vi "Test Set Class.vi"(8 "error in (no error)":errorcluster, 11 "TestCase in":refnum<class "Test FP.lvclass">) -> (0 "error out":errorcluster, 3 "TestCase out":refnum<class "Test FP.lvclass">)   [LabVIEW 2020, in "Test FP.lvclass"]
uses:
  Test FP.lvclass
  Classes/Implementations/Osciloscope/Osciloscope.lvclass
  <vilib>/addons/_JKI Toolkits/VI Tester/TestCase.llb/TestCase.lvclass
  C:/Program Files (x86)/National Instruments/LabVIEW 2020/vi.lib/addons/_JKI Toolkits/VI Tester/TestCase.llb/TestCase.lvclass
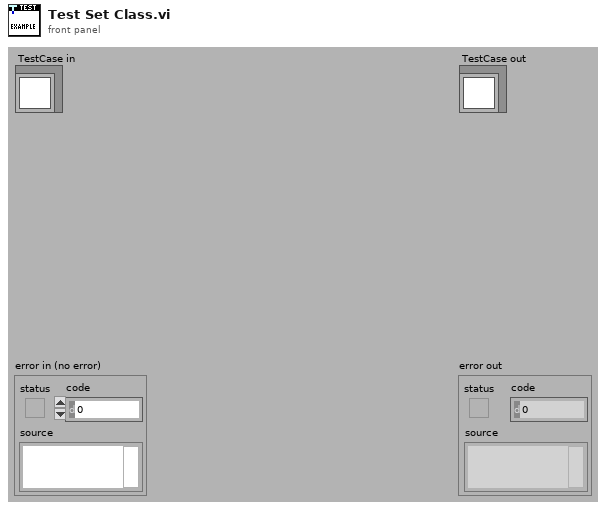
[diagram p1: front panel]
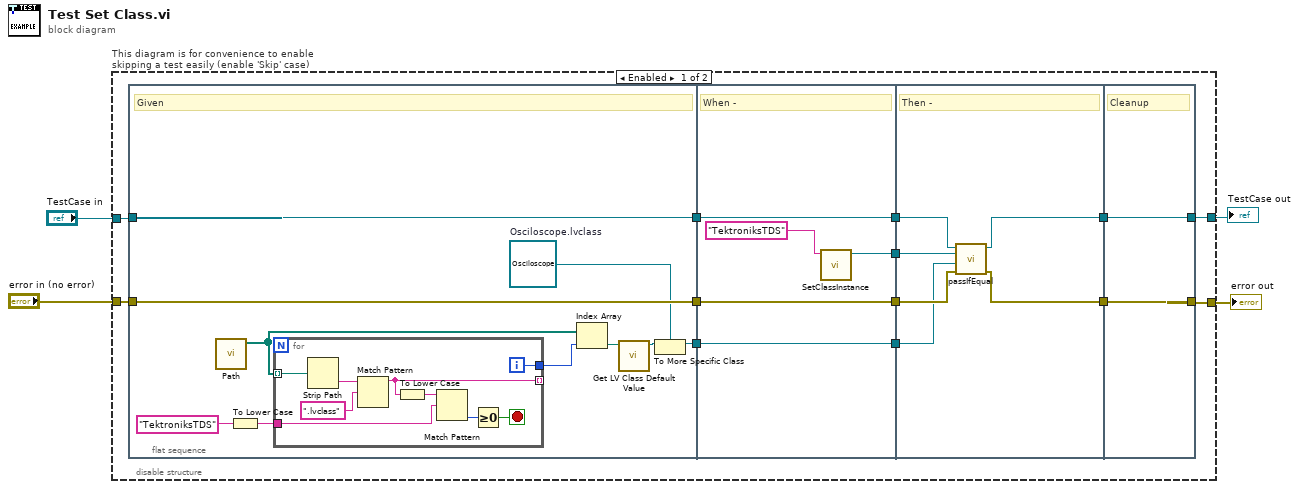
[diagram p0: block diagram]
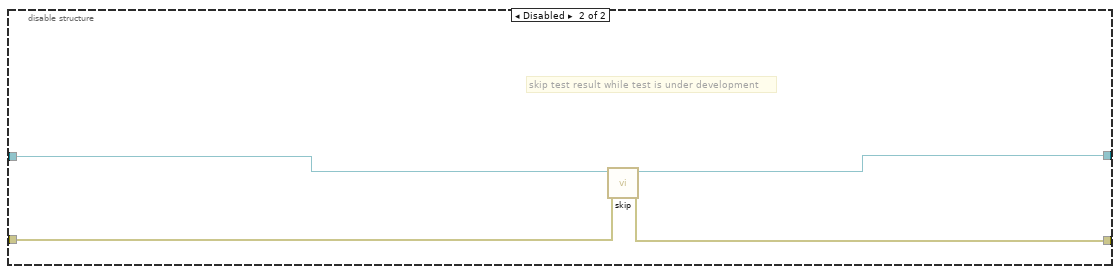
[diagram p2: hidden frame]
diagram:
  n1 = disable-structure "This diagram is for convenience to enable skipping a test easily (enable 'Skip' case)" shown="Enabled" {
    disable-tunnel: "TestCase in" -> [w11 w53]
    disable-tunnel: [w9 w51] -> w1
    disable-tunnel: [w8 w52] -> w3
    disable-tunnel: "error in (no error)" -> [w10 w50]
    frame Enabled {
      n2 = flat-sequence {
        tunnel: w10 -> [w26]
        tunnel: w11 -> [w27]
        tunnel: [w27] -> w17
        tunnel: [w26] -> w16
        tunnel: [w18] -> w5
        tunnel: [w41] -> w15
        tunnel: [w40] -> w14
        tunnel: w17 -> [w41]
        tunnel: w16 -> [w40]
        tunnel: [w39] -> w7
        tunnel: [w38] -> w6
        tunnel: w5 -> [w38]
        tunnel: [w46] -> w13
        tunnel: [w44] -> w12
        tunnel: w15 -> [w47]
        tunnel: w14 -> [w45]
        tunnel: w7 -> [w43]
        tunnel: w6 -> [w42]
        tunnel: [w48] -> w8
        tunnel: [w49] -> w9
        tunnel: w13 -> [w49]
        tunnel: w12 -> [w48]
        frame #0 {
          w21 = refnum<class "Osciloscope.lvclass"> refnum  # Osciloscope.lvclass
          # "Given"
          n3 = call "Path.vi"() -> ("All Files in Dir"=w19:path[])  [unwired: 11 in]
          n4 = To Lower Case(string="TektroniksTDS") -> (all lower case string=w25:string)
          n5 = for {
            tunnel: w19 -> [w35] mode=indexing
            tunnel: [w33] -> _ mode=indexing
            tunnel: w25 -> [w31]
            tunnel: [w28] -> w24
            i -> [w28]
            stop <- w30 stop-if-true
            n6 = Strip Path(path=w35) -> (name=w34:string)  [unwired: 1 out]
            n7 = Match Pattern(string=w34, regular expression=".lvclass") -> (before substring=w33:string)  [unwired: 1 in, 3 out]
            n8 = To Lower Case(string=w33) -> (all lower case string=w32:string)
            n9 = Match Pattern(string=w32, regular expression=w31) -> (offset past match=w29:i32)  [unwired: 1 in, 3 out]
            n10 = Greater Or Equal To 0?(x=w29) -> (x >= 0?=w30:bool)
          }
          n11 = Index Array(array=w19, index=w24) -> (element=w22:path)
          n12 = call <vilib>:"Get LV Class Default Value.vi"("class path"=w22) -> ("object"=w23:refnum<class>)  [unwired: 9 in, 1 out]
          n13 = To More Specific Class(target class=w21, reference=w23) -> (specific class reference=w18:refnum<class "Osciloscope.lvclass">)  [unwired: 1 in, 1 out]
        }
        frame #1 {
          # "When -"
          n14 = call "SetClassInstance.vi"("OsciloscopioName"="TektroniksTDS" ("string")) -> ("specific class reference"=w39:refnum<class "Osciloscope.lvclass">)  [unwired: 10 in]
        }
        frame #2 {
          # "Then -"
          n15 = call-dynamic "passIfEqual.vi"("error in (no error)"=w45, "y"=w42, "x"=w43, "TestCase in"=w47) -> ("error out"=w44:errorcluster, "TestCase out"=w46:refnum<class "Test FP.lvclass">)  [unwired: 6 in]
        }
        frame #3 {
          # "Cleanup"
        }
      }
    }
    frame Disabled {
      # "skip test result while test is under development"
      n16 = call <vilib>:"skip.vi"("error in (no error)"=w50, "TestCase in"=w53) -> ("error out"=w52:errorcluster, "TestCase out"=w51:refnum<class "Test FP.lvclass">)  [unwired: 8 in]
    }
  }
  "error out" <- w3
  "TestCase out" <- w1
